vi "Generate Leafs Item.vi"(6 "File Symbol Index In":i32, 8 "error in (no error)":errorcluster, 9 "Tree Item In":T1, 10 "Root Tag In":string, 11 "Tree Data Folder In":refnum<class "Tree Data Folder.lvclass">) -> (0 "error out":errorcluster, 1 "Leafs Item Out":T1[](array[typedef]), 3 "Tree Data Folder Out":refnum<class "Tree Data Folder.lvclass">)   [LabVIEW 2019, in "Tree Data Folder.lvclass"]
uses:
  Tree Data Folder.lvclass
  Tree/Type Def/Tree Item.ctl
  C:/Users/iio/Desktop/NTHU Brain Center/General Purpose/Classes/Ancestor/Front Panel Container/Tree/Composite Tree Data/Composite Tree Data.lvclass
  Tree Data Folder.lvclass/Tree Data Folder.ctl
  Composite Tree Data/Composite Tree Data.lvclass/Composite Tree Data.ctl
  Composite Tree Data/Protected Data/Read Sub Nodes.vi
  Polymorphic VIs/Tree Converter/BFS Index To Tag.vi
  Tree Data/Tree Data.lvclass
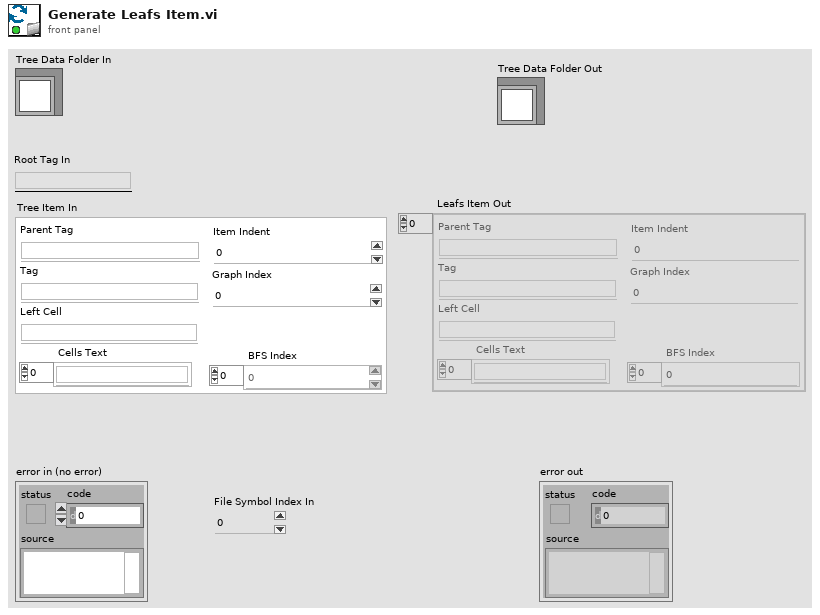
[diagram p1: front panel]
types:
  T1 = typedef "Tree Item.ctl" = cluster{"Parent Tag":string, "Tag":string, "Left Cell":string, "Cells Text":string[], "BFS Index":i32[], "Graph Index":i32, "Item Indent":i32}
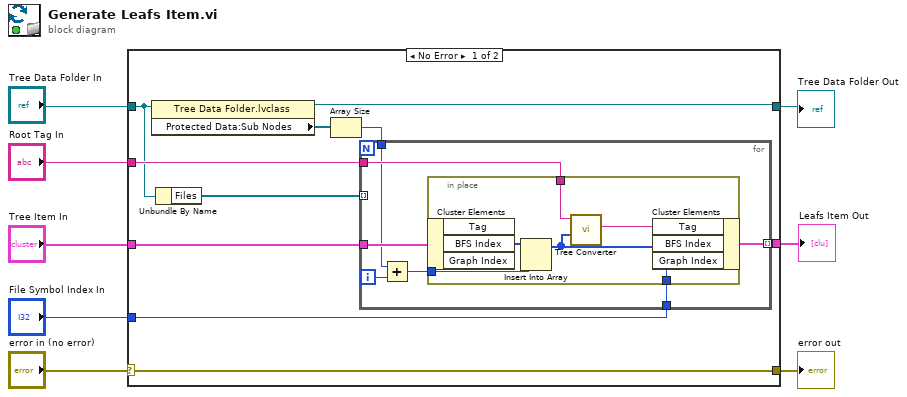
[diagram p0: block diagram]
diagram:
  n1 = case shown="No Error" "error in (no error)" {
    selector: "error in (no error)" -> [w18 w33]
    tunnel: [w18 w33] -> w7
    tunnel: [w11 w32] -> w2
    tunnel: "Tree Data Folder In" -> [w12 w32]
    tunnel: [w16 _] -> w6
    tunnel: "Tree Item In" -> [w15 _]
    tunnel: "Root Tag In" -> [w14 _]
    tunnel: "File Symbol Index In" -> [w13 _]
    frame No Error {
      n2 = property class="Tree Data Folder.lvclass"(reference=w12) -> (reference out=w11:refnum<class "Tree Data Folder.lvclass">, "Protected Data:Sub Nodes"=w10:refnum<class "Tree Data.lvclass">[])  [unwired: 1 in, 1 out]
      n3 = Unbundle By Name(w12) -> ("Files"=w17:refnum<class "Tree Data File.lvclass">[])
      n4 = Array Size(array=w10) -> (size(s)=w9:i32)
      n5 = for {
        tunnel: w17 -> [_] mode=indexing
        tunnel: [w24] -> w16 mode=indexing
        tunnel: w15 -> [w25]
        tunnel: w14 -> [w23]
        tunnel: w13 -> [w22]
        tunnel: w9 -> [w19]
        i -> [w20]
        n6 = Add(x=w19, y=w20) -> (x+y=w21:i32)
        n7 = in-place {
          in-place-border: w21 -> [w30]
          in-place-border: w23 -> [w27]
          in-place-border: w22 -> [w26]
          n8 = in-place-cluster #1(w25) -> ("BFS Index"=w31:i32[])  [unwired: 2 out]
          n9 = Insert Into Array(array=w31, new element=w30) -> (w28:i32[])  [unwired: 1 in]
          n10 = call-poly "Tree Converter.vi"("BFS Index In"=w28, "Root Tag In"=w27) -> ("Tag Out"=w29:string)  [unwired: 9 in]
          n11 = in-place-cluster #1("Tag"=w29, "BFS Index"=w28, "Graph Index"=w26) -> (w24:T1)
        }
      }
    }
    frame Error {
    }
  }
  "error out" <- w7
  "Leafs Item Out" <- w6
  "Tree Data Folder Out" <- w2
